vi "SENS_AVER_COUN.vi"(0 "VISA IN":refnum<visa-resource-name>, 2 "AVG":i32, 5 "error in":errorcluster, 7 "Channel":i32) -> (14 "VISA Out":refnum<visa-resource-name>, 19 "error out":errorcluster)   [LabVIEW 2018, in "PNA-X.lvlib"]
doc: "SENSe<cnum>:AVERage:COUNt <num> \n1619\n\n(Read-Write) Sets the number of measurement sweeps to combine for an average. Must also set \nSENS:AVER[:STATe] ON \nParameters \n<cnum> Any existing channel number; if unspecified, value is set to 1. \n<num> Number of measurement sweeps to average. Choose any number between 1 \nand 65536 (2^16). \nExamples SENS:AVER:COUN 999 \nsense2:average:count 73 \nQuery Syntax SENSe<cnum>:AVERage:COUNt? \nReturn Type Numeric \nDefault 1"
uses:
  PNA-X.lvlib
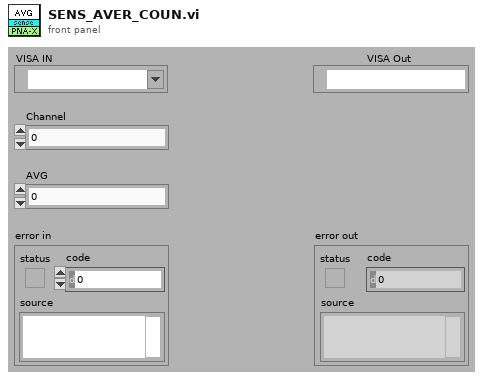
[diagram p1: front panel]
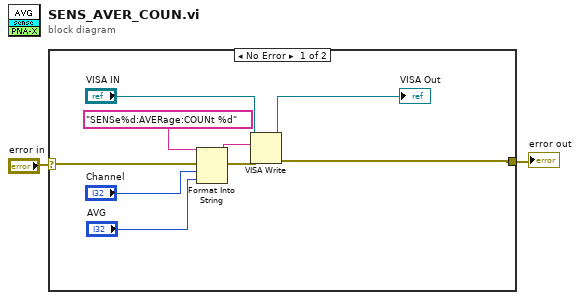
[diagram p0: block diagram]
diagram:
  n1 = case shown="No Error" "error in" {
    selector: "error in" -> [w11 w12]
    tunnel: [w7 w12] -> w1
    frame No Error {
      n2 = Format Into String(format string="SENSe%d:AVERage:COUNt %d" ("Cmdline"), error in=w11, "Channel", "AVG") -> (resulting string=w9:string, error out=w10:errorcluster)  [unwired: 1 in]
      n3 = VISA Write(VISA resource name="VISA IN", write buffer=w9, error in (no error)=w10) -> (VISA resource name out=→"VISA Out":refnum<visa-resource-name>, error out=w7:errorcluster)  [unwired: 1 out]
    }
    frame Error {
    }
  }
  "error out" <- w1
